vi "搜索元素索引.vi"(1 "搜索值":i32, 3 "数组":i32[][](array[numeric])) -> (0 "索引簇":cluster{i32, i32}[](array[cluster]))   [LabVIEW 2020]
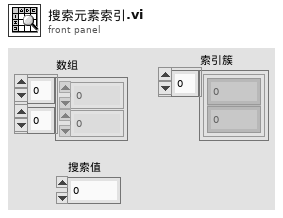
[diagram p1: front panel]
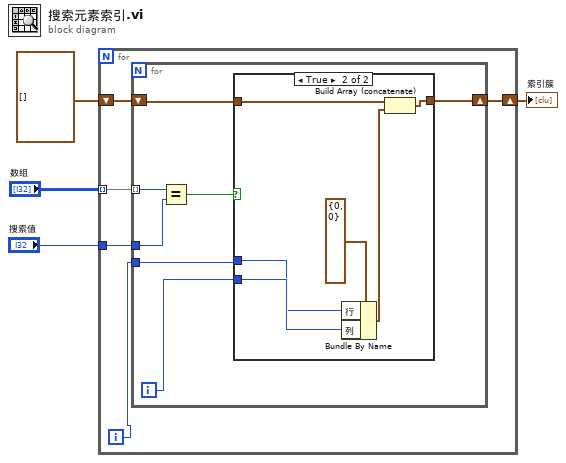
[diagram p0: block diagram]
diagram:
  n1 = for {
    tunnel: "数组" -> [w9] mode=indexing
    shift-right: [w8] -> w1
    shift-left: cluster{"行":i32, "列":i32}[] [] -> [w7]
    tunnel: "搜索值" -> [w5]
    i -> [w6]
    n2 = for {
      tunnel: w9 -> [w16] mode=indexing
      shift-right: [w11] -> w8
      shift-left: w7 -> [w12]
      tunnel: w6 -> [w13]
      tunnel: w5 -> [w10]
      i -> [w14]
      n3 = Equal?(x=w16, y=w10) -> (x = y?=w15:bool)
      n4 = case shown="True" w15 {
        tunnel: w14 -> [_ w19]
        tunnel: w13 -> [_ w18]
        tunnel: w12 -> [w17 w23]
        tunnel: [w17 w22] -> w11
        frame False {
        }
        frame True {
          n5 = Bundle By Name(cluster=cluster{"行":i32, "列":i32} {"行"=0, "列"=0}, "行"=w18, "列"=w19) -> (w21:cluster{"行":i32, "列":i32})
          n6 = Build Array (concatenate)(w23, w21) -> (w22:cluster{"行":i32, "列":i32}[])
        }
      }
    }
  }
  "索引簇" <- w1
